vi "_Error-FunctionNotAvailable.vi"() -> (0 "error out":errorcluster)   [LabVIEW 2020, in "hse-db-ado.lvlib" / "DB-ADO.lvclass"]
doc: "____\nHAMPEL SOFTWARE ENGINEERING v1.4.0 (2023-12-19 09:52)"
uses:
  DB-ADO.lvclass
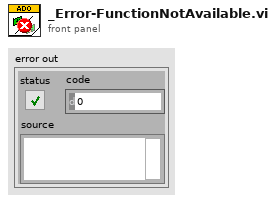
[diagram p1: front panel]
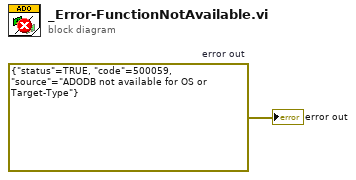
[diagram p0: block diagram]
diagram:
  w1 = errorcluster {"status"=TRUE, "code"=500059, "source"="ADODB not available for OS or Target-Type"}  # error out
  "error out" <- w1
